vi "Monitor Aurora Link.vi"(8 "error in (no error)":errorcluster, 11 "niUsrpRio Sessions (In)":T1[](array[typedef]) {"Daughterboard Clock Rate" format="%#.3pHz"; "FPGA Data Clock Rate" format="%#.3pHz"; "Data Clock Rate" format="%#.3pHz"; "Characterization Data"."Frequencies [Hz]" format="%#_6p"; "EEPROM Characterization Header"."Pointer to Device Data Header" format="%x"; "EEPROM Characterization Header"."Checksum" format="%x"; "Device Data Header"."Pointer to Characterization Data" format="%x"; "Device Data Header"."Checksum" format="%x"; "EEPROM Header"."Pointer to User Header" format="%x"; "EEPROM Header"."Pointer to Factory Header" format="%x"; "EEPROM Header"."Product Code" format="%x"; "EEPROM Header"."Checksum" format="%x"}) -> (0 "error out":errorcluster, 1 "niUsrpRio Sessions (Out)":T1[](array[typedef]) {"Daughterboard Clock Rate" format="%#.3pHz"; "FPGA Data Clock Rate" format="%#.3pHz"; "Data Clock Rate" format="%#.3pHz"; "Characterization Data"."Frequencies [Hz]" format="%#_6p"; "EEPROM Characterization Header"."Pointer to Device Data Header" format="%x"; "EEPROM Characterization Header"."Checksum" format="%x"; "Device Data Header"."Pointer to Characterization Data" format="%x"; "Device Data Header"."Checksum" format="%x"; "EEPROM Header"."Pointer to User Header" format="%x"; "EEPROM Header"."Pointer to Factory Header" format="%x"; "EEPROM Header"."Product Code" format="%x"; "EEPROM Header"."Checksum" format="%x"}, 2 "FIFO USRP >>> HSDIO":u32, 3 "Overflow":bool)   [LabVIEW 2016]
uses:
  <instrlib>/niUsrpRio/Config/v1/Host/Public/niUsrpRio Session.ctl
  <instrlib>/_niInstr/Register Bus/v0/Host/Public/Register Bus Session.ctl
  <instrlib>/_niInstr/Register Bus/v0/Host/Private/Session Data.ctl
  <instrlib>/niUsrpRio/Config/v1/Host/Private/DB Queue Reference.ctl
  <instrlib>/niUsrpRio/Config/v1/Host/Private/Daughterboard Data.ctl
  <instrlib>/niUsrpRio/Config/v1/Host/Private/ATR state data.ctl
  <instrlib>/niUsrpRio/Config/v1/Host/Private/Antenna Configuration.ctl
  <instrlib>/niUsrpRio/Config/v1/Host/Private/CPLD Power Mode.ctl
  <instrlib>/niUsrpRio/Config/v1/Host/Public/EEPROM Header.ctl
  <instrlib>/niUsrpRio/Config/v1/Host/Public/EEPROM Device Data Header.ctl
  <instrlib>/niUsrpRio/Config/v1/Host/Public/EEPROM Characterization Header.ctl
  <instrlib>/niUsrpRio/Config/v1/Host/Public/Characterization Data.ctl
  <instrlib>/niUsrpRio/Config/v1/Host/Public/IQ Imbalance.ctl
  <instrlib>/_niInstr/Register Bus/v0/Host/niInstr Register Bus v0 Host.lvlib
  <instrlib>/niUsrpRio/Config/v1/Host/niUsrpRio Config v1 Host.lvlib
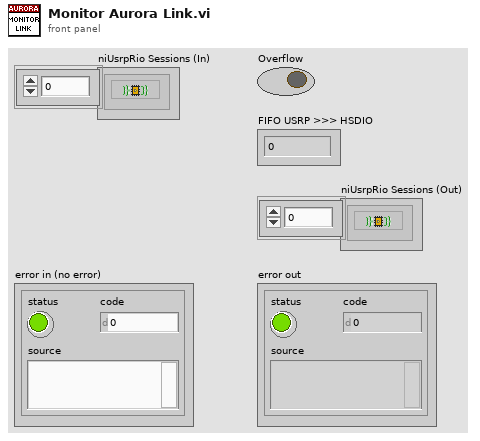
[diagram p1: front panel]
types:
  T1 = typedef "niUsrpRio Config v1 Host.lvlib/niUsrpRio Session.ctl" = cluster{"FPGA Interface":refnum<k20>, "RIO Interface Number":u32, "Data Clock Rate":u32, "FPGA Data Clock Rate":u32, "Global Settings Register Bus":T2, "Radio 0 Settings Register Bus":T2, "Radio 1 Settings Register Bus":T2, "Radio Settings Bus Semaphore":T3, "DB Queues":T4[], "Characterization Data Valid?":bool, "EEPROM Header":T5, "Device Data Header":T6, "EEPROM Characterization Header":T7, "Characterization Data":T8[], "FPGA Current Version":u32, "FPGA Oldest Compatible Version":u32, "Fixed Logic Current Version":u32, "Fixed Logic Oldest Compatible Version":u32, "FPGA Radio Settings Bus Current Version":u32, "FPGA Radio Settings Bus Oldest Compatible Version":u32, "FPGA Board Config Current Version":u32, "FPGA Board Config Oldest Compatible Version":u32, "Daughterboard Clock Rate":u32, "daughterboard configuration session handles":u64[]}
  T2 = typedef "niInstr Register Bus v0 Host.lvlib/Register Bus Session.ctl" = refnum<queue>
  T3 = typedef "Semaphore RefNum" = refnum<k1>
  T4 = typedef "niUsrpRio Config v1 Host.lvlib/DB Queue Reference.ctl" = refnum<queue>
  T5 = typedef "niUsrpRio Config v1 Host.lvlib/EEPROM Header.ctl" = cluster{"Checksum":u32, "Product Code":u16, "Hardware Current Version":u16, "Hardware Oldest Compatible Version":u16, "EEPROM Map Current Version":u16, "EEPROM Map Oldest Compatible Version":u16, "User Password":string, "Pointer to Factory Header":u32, "Pointer to User Header":u32, "Recommended Interval":u16, "Number of Reserved Bytes":i32, "Number of Daughterboards":u8, "Daughterboard IDs":u16[], "Daughterboard Serial Numbers":string[]}
  T6 = typedef "niUsrpRio Config v1 Host.lvlib/EEPROM Device Data Header.ctl" = cluster{"Checksum":u32, "Number of Channels":u8, "Number of Gain Settings":u16[], "Pointer to Characterization Data":u32[], "Number of Reserved Bytes":i32, "Number of Frequencies":u16[]}
  T7 = typedef "niUsrpRio Config v1 Host.lvlib/EEPROM Characterization Header.ctl" = cluster{"Checksum":u32, "Date":timestamp, "Temperature":sgl, "Misc. Info":string, "Pointer to Device Data Header":u32, "Number of Reserved Bytes":i32}
  T8 = typedef "niUsrpRio Config v1 Host.lvlib/Characterization Data.ctl" = cluster{"Gains[dB]":dbl[], "Frequencies [Hz]":dbl[], "IQ Imbalance Table":T9[], "Measured Gains[dB]":dbl[][]}
  T9 = typedef "niUsrpRio Config v1 Host.lvlib/IQ Imbalance.ctl" = cluster{"Gain Imbalance [linear]":dbl, "Phase Imbalance [radians]":dbl, "Offset":cdb}
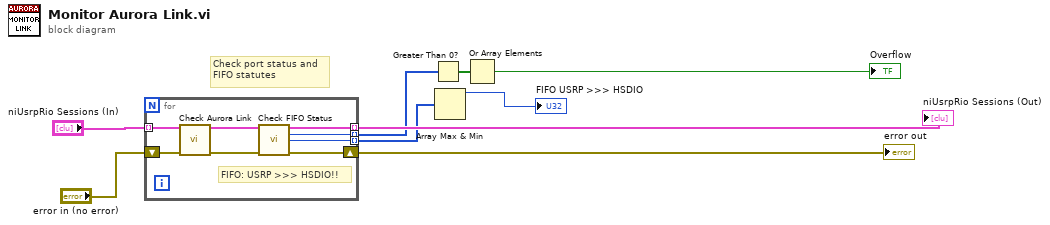
[diagram p0: block diagram]
diagram:
  # "Check port status and\nFIFO statutes"
  n1 = for {
    shift-right: [w14] -> w7
    shift-left: "error in (no error)" -> [w17]
    tunnel: "niUsrpRio Sessions (In)" -> [w16] mode=indexing
    tunnel: [w12] -> w9 mode=indexing
    tunnel: [w11] -> w2 mode=indexing
    tunnel: [w10] -> w4 mode=indexing
    # "FIFO: USRP >>> HSDIO!!"
    n2 = call "Check Aurora Link.vi"("niUsrpRio Session"=w16, "error in"=w17) -> ("niUsrpRio Session (out)"=w13:T1, "error out"=w15:errorcluster)  [unwired: 11 in, 1 out]
    n3 = call "Check FIFO Status.vi"("niUsrpRio Session in"=w13, "Error In"=w15) -> ("niUsrpRio Session out"=w12:T1, "rx.number of fifo overflows"=w11:u32, "F0"=w10:u32, "Error Out"=w14:errorcluster)  [unwired: 9 in, 1 out]
  }
  "niUsrpRio Sessions (Out)" <- w9
  "error out" <- w7
  n4 = Greater Than 0?(x=w2) -> (x > 0?=w1:bool[])
  n5 = Array Max & Min(array=w4) -> (max value=→"FIFO USRP >>> HSDIO":u32)  [unwired: 3 out]
  n6 = Or Array Elements(Boolean array=w1) -> (logical OR=→"Overflow":bool)
